vi "Add_Module.vi"(8 "Error In":errorcluster, 11 "Module Name":string) -> (0 "error out":errorcluster)   [LabVIEW 2015, in "Generic Module Library.lvlib"]
uses:
  Generic Module Library.lvlib
panel:
  out "Module Name":string
  # "THERE'S NO RUN BUTTON??\n\nInstead of opening this VI and running it. Right click this VI from within a LabVIEW project and select \"Run\". This will cause the VI to run and allow you to give your new module a name."
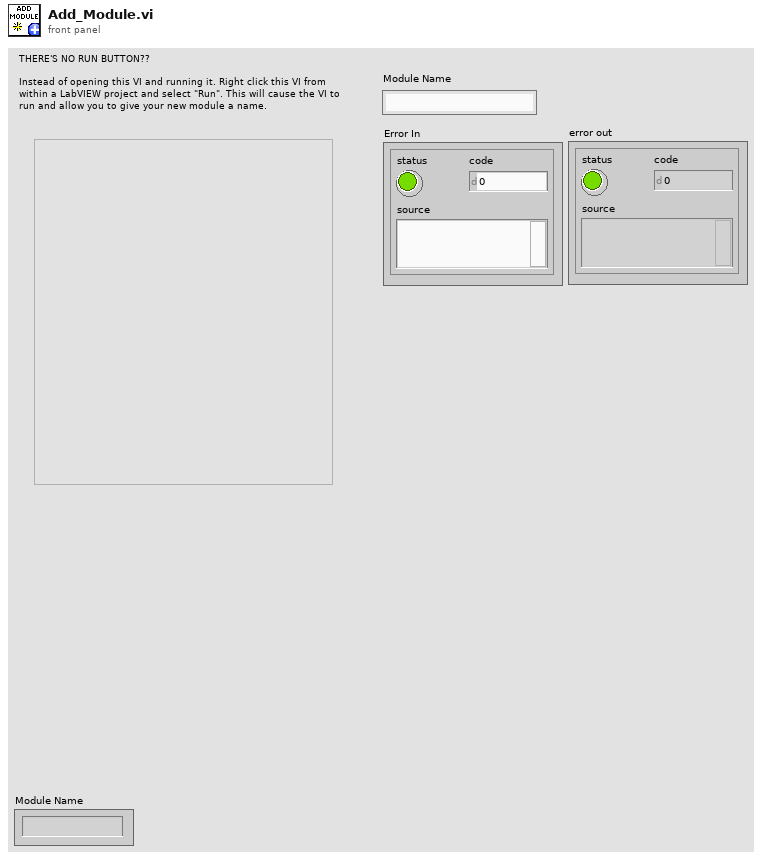
[diagram p1: front panel]
types:
  T1 = enum32{"Invalid", "Standard", "Closed", "Hidden", "Minimized", "Maximized"}
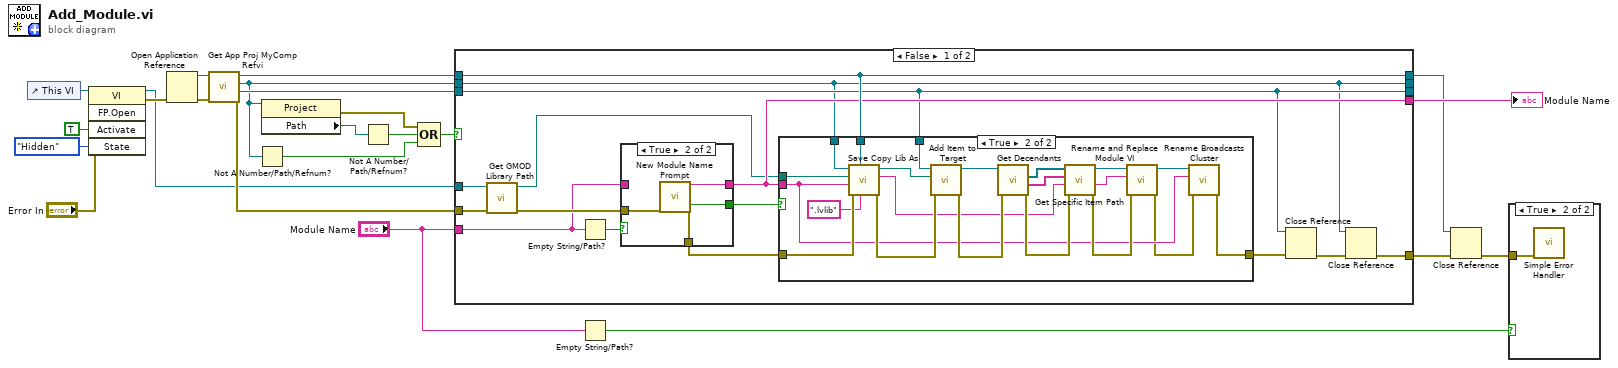
[diagram p0: block diagram]
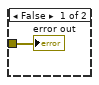
[diagram p2: hidden frame]
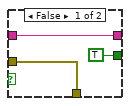
[diagram p3: hidden frame]
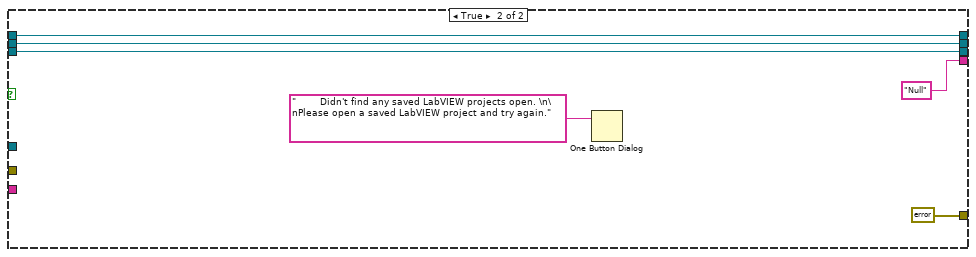
[diagram p5: hidden frame]
diagram:
  n1 = control-ref of="This VI"() -> (w19:refnum<vi>)
  n2 = invoke class="VI" method="FP.Open"(reference=w19, error in="Error In", "Activate"=TRUE ("Activate?"), "State"=T1."Hidden") -> (reference out=w4:refnum<vi>, error out=w22:errorcluster)  [unwired: 1 in, 3 out]
  n3 = Open Application Reference(8:w22) -> (0:w23:errorcluster, 3:w18:refnum<vi>)  [unwired: 3 in]
  n4 = call "Get App Proj MyComp Refvi.vi"("error in (no error)"=w23, "Application in"=w18) -> ("error out"=w16:errorcluster, "My Computer"=w15:refnum<vi>, "Project Refnum"=w14:refnum<vi>, "Application out"=w17:refnum<vi>)  [unwired: 6 in]
  n5 = Not A Number/Path/Refnum?(number/path/refnum=w14) -> (NaN/Path/Refnum?=w11:bool)
  n6 = property class="Project"(reference=w14) -> (error out=w9:errorcluster, "Path"=w5:path)  [unwired: 1 in, 1 out]
  n7 = Not A Number/Path/Refnum?(number/path/refnum=w5) -> (NaN/Path/Refnum?=w12:bool)
  n8 = Compound Arithmetic op=OR(w9, w12, w11) -> (w13:bool)
  n9 = case shown="False" w13 {
    tunnel: w17 -> [w35 w71]
    tunnel: w16 -> [w29 _]
    tunnel: w15 -> [w33 w73]
    tunnel: w14 -> [w31 w72]
    tunnel: [w31 w72] -> _
    tunnel: [w35 w71] -> w7
    tunnel: [w33 w73] -> _
    tunnel: [w32 errorcluster {"status"=FALSE, "code"=0, "source"=""} ("error out")] -> w6
    tunnel: [w34 "Null" ("Name")] -> w10
    tunnel: w4 -> [w30 _]
    tunnel: "Module Name" -> [w24 _]
    frame False {
      n10 = call "Get GMOD Library Path.vi"("error in (no error)"=w29, "VI in"=w30) -> ("error out"=w28:errorcluster, "appended path"=w25:path)  [unwired: 8 in]
      n11 = Empty String/Path?(string/path=w24) -> (empty?=w26:bool)
      n12 = case shown="True" w26 {
        tunnel: [w40 w45] -> w38
        tunnel: [w41 w44] -> w34
        tunnel: w28 -> [w40 w43]
        tunnel: [TRUE ("OK") w42] -> w27
        tunnel: w24 -> [w41 _]
        frame False {
        }
        frame True {
          n13 = call "New Module Name Prompt.vi"("error in (no error)"=w43) -> ("Name"=w44:string, "OK"=w42:bool, "error out"=w45:errorcluster)  [unwired: 16 in]
        }
      }
      n14 = case shown="True" w27 {
        tunnel: [w46 w52] -> w37
        tunnel: w34 -> [_ w54]
        tunnel: w35 -> [_ w48]
        tunnel: w33 -> [_ w66]
        tunnel: w38 -> [w46 w65]
        tunnel: w25 -> [_ w49]
        tunnel: w31 -> [_ w47]
        frame False {
        }
        frame True {
          n15 = call "Save Copy Lib As.vi"("Extension"=".lvlib", "Application in"=w48, "error in (no error)"=w65, "New Name"=w54, "Path to Lib Being Copied"=w49, "Project In"=w47) -> ("error out"=w64:errorcluster, "New Module/Lib Name"=w55:string, "New Path"=w67:path)  [unwired: 2 in, 1 out]
          n16 = call "Add Item to Target.vi"("error in (no error)"=w64, "New Item Path"=w67, "TargetRef In"=w66) -> ("error out"=w56:errorcluster, "TargetRef Out"=w57:refnum<vi>)  [unwired: 7 in]
          n17 = call "Get Decendants.vi"("error in (no error)"=w56, "TargetRef in"=w57) -> ("error out"=w61:errorcluster, "Names"=w62:string[], "Decendant References"=w63:refnum<vi>[])  [unwired: 6 in, 1 out]
          n18 = call "Get Specific Item Path.vi"("error in (no error)"=w61, "Item to find"=w55, "Names"=w62, "Decendant References"=w63) -> ("error out"=w60:errorcluster, "Item Name"=w59:string, "Item Reference"=w51:refnum<vi>)  [unwired: 4 in, 1 out]
          n19 = call "Rename and Replace Module VI.vi"("error in (no error)"=w60, "New Module/Lib Name"=w59, "ProjectItem In"=w51) -> ("error out"=w53:errorcluster, "ProjectItem Out"=w50:refnum<vi>)  [unwired: 5 in, 2 out]
          n20 = call "Rename Broadcasts Cluster.vi"("error in (no error)"=w53, "Name"=w54, "TargetRef in"=w50) -> ("error out"=w52:errorcluster)  [unwired: 8 in]
        }
      }
      n21 = Close Reference(reference=w33, error in (no error)=w37) -> (error out=w36:errorcluster)
      n22 = Close Reference(reference=w31, error in (no error)=w36) -> (error out=w32:errorcluster)
    }
    frame True {
      n23 = One Button Dialog(message="        Didn't find any saved LabVIEW projects open. \n\nPlease open a saved LabVIEW project and try again.") -> ()  [unwired: 1 in, 1 out]
    }
  }
  "Module Name" <- w10
  n24 = Empty String/Path?(string/path="Module Name") -> (empty?=w1:bool)
  n25 = Close Reference(reference=w7, error in (no error)=w6) -> (error out=w8:errorcluster)
  n26 = case shown="True" w1 {
    tunnel: w8 -> [w74 w75]
    frame False {
      "error out" <- w74
    }
    frame True {
      n27 = call <vilib>:"Simple Error Handler.vi"("error in (no error)"=w75) -> ()  [unwired: 4 in, 5 out]
    }
  }
